vi "poly_asynch_wait_stop.vi"(8 "error in":errorcluster, 10 "asynch wait ref in":T2) -> (0 "error out":errorcluster, 2 "notifier":T1)   [LabVIEW 2015, in "_timing_tools_polys.lvlib"]
uses:
  _timing_tools_polys.lvlib
  asynch_wait_ref.ctl
  boolean_notifier.ctl
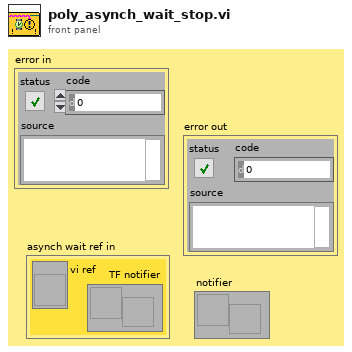
[diagram p1: front panel]
types:
  T1 = typedef "_timing_tools_polys.lvlib/boolean_notifier.ctl" = refnum<notifier>
  T2 = typedef "_timing_tools_polys.lvlib/asynch_wait_ref.ctl" = cluster{"vi ref":refnum<vi>, "TF notifier":T1}
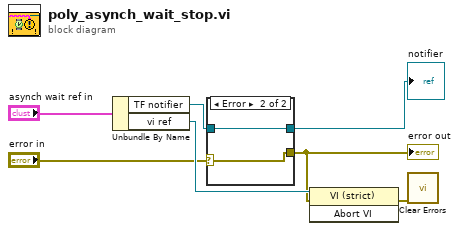
[diagram p0: block diagram]
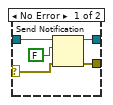
[diagram p2: hidden frame]
diagram:
  n1 = Unbundle By Name("asynch wait ref in") -> ("TF notifier"=w4:T1, "vi ref"=w6:refnum<vi>)
  n2 = case shown="Error" "error in" {
    selector: "error in" -> [w8 w13]
    tunnel: w4 -> [w12 w14]
    tunnel: [w11 w13] -> w1
    tunnel: [w9 w14] -> w2
    frame No Error {
      n3 = Send Notification(notification=FALSE, notifier=w12, error in (no error)=w8) -> (notifier out=w9:T1, error out=w11:errorcluster)
    }
    frame Error {
    }
  }
  "error out" <- w1
  "notifier" <- w2
  n4 = invoke class="VI (strict)" method="Abort VI"(reference=w6, error in=w1) -> (error out=w5:errorcluster)  [unwired: 1 in, 2 out]
  n5 = call <vilib>:"Clear Errors.vi"("error in (no error)"=w5) -> ()  [unwired: 5 in, 2 out]
